vi "RT_DAC1.vi"() -> ()   [LabVIEW 2018]
uses:
  <vilib>/FPGAPlugInAG/myRIO-1900/niLvFpga_Open_myRIO-1900.vi
  <vilib>/rvi/interface/common/dynamic/niFpgaDynamicAddResources.vi
  <vilib>/Utility/error.llb/Error Cluster From Error Code.vi
  <vilib>/rvi/errors/niLvFpgaAdjustHostInterfaceError.vi
  <vilib>/FPGAPlugInAG/Dynamic/niLvFpga_Close_Dynamic.vi
  <vilib>/rvi/interface/nirviOpenFPGA/nirviOpenFPGA.xnode
  FPGA Bitfiles/WattBalanceRev1_FPGATarget_FPGASPI2_21rs6YSGst0.lvbitx
  <vilib>/rvi/interface/nirviReadWriteControl/nirviReadWriteControl.xnode
  <vilib>/rvi/interface/nirviCloseFPGA/nirviCloseFPGA.xnode
  NiFpgaLv.dll
  <vilib>/rvi/interface/Simulation/niFpgaSimulationCallBeginRW.vi
panel:
  in  "Stop Button":bool
  in  "voltage":dbl
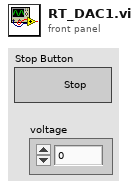
[diagram p1: front panel]
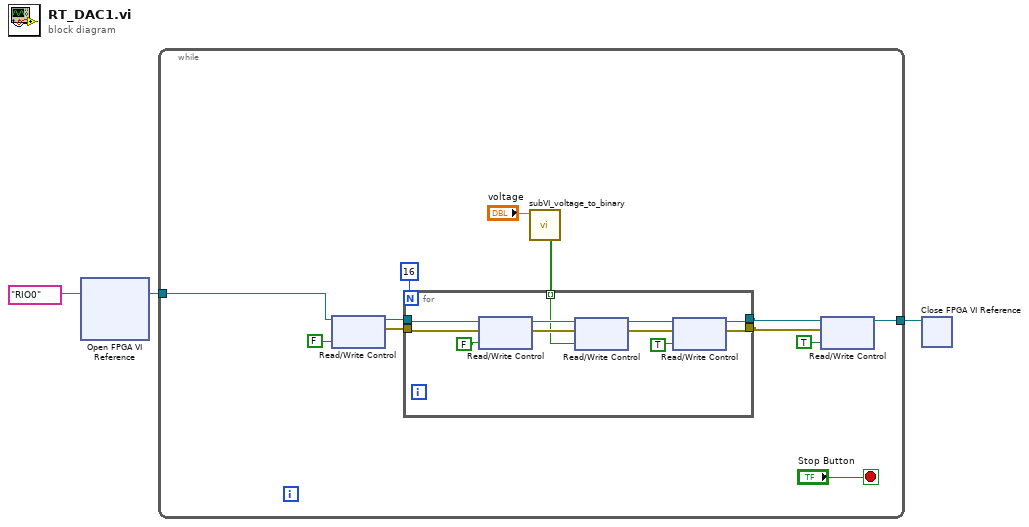
[diagram p0: block diagram]
diagram:
  n1 = xnode "Open FPGA VI Reference"("resource name"=tag "RIO0") -> ("FPGA VI Reference Out"=w2:refnum<k20>)  [unwired: 1 in, 1 out]
  n2 = while {
    tunnel: w2 -> [w7]
    tunnel: [w4] -> w1
    stop <- "Stop Button" stop-if-true
    n3 = xnode "Read/Write Control"("FPGA VI Reference In"=w7, "CS"=FALSE) -> ("FPGA VI Reference Out"=w12:refnum<k20>, "error out"=w11:errorcluster)  [unwired: 1 in]
    n4 = call "subVI_voltage_to_binary.vi"("voltage"="voltage") -> ("binary"=w5:bool[])  [unwired: 10 in]
    n5 = for {
      N: 16 -> [_]
      tunnel: w12 -> [w22]
      tunnel: w11 -> [w21]
      tunnel: [w19] -> w14
      tunnel: [w18] -> w13
      tunnel: w5 -> [w20] mode=indexing
      n6 = xnode "Read/Write Control"("FPGA VI Reference In"=w22, "error in"=w21, "CLK2"=FALSE ("CLK")) -> ("FPGA VI Reference Out"=w26:refnum<k20>, "error out"=w25:errorcluster)
      n7 = xnode "Read/Write Control"("FPGA VI Reference In"=w26, "error in"=w25, "MOSI2"=w20) -> ("FPGA VI Reference Out"=w24:refnum<k20>, "error out"=w23:errorcluster)
      n8 = xnode "Read/Write Control"("FPGA VI Reference In"=w24, "error in"=w23, "CLK2"=TRUE) -> ("FPGA VI Reference Out"=w19:refnum<k20>, "error out"=w18:errorcluster)
    }
    n9 = xnode "Read/Write Control"("FPGA VI Reference In"=w14, "error in"=w13, "CS"=TRUE) -> ("FPGA VI Reference Out"=w4:refnum<k20>)  [unwired: 1 out]
  }
  n10 = xnode "Close FPGA VI Reference"("FPGA VI Reference In"=w1) -> ()  [unwired: 1 in, 1 out]
